vi "randImg.vi"(8 "error in (no error)":errorcluster) -> (0 "error out":errorcluster, 2 "2D Picture":picture, 3 "string out (base64-encoded)":string)   [LabVIEW 2018]
uses:
  abde8a46-2864-4d9c-bf4c-91a7911b97bf.vi
  <vilib>/wsapi/NI_WebServices.lvlib
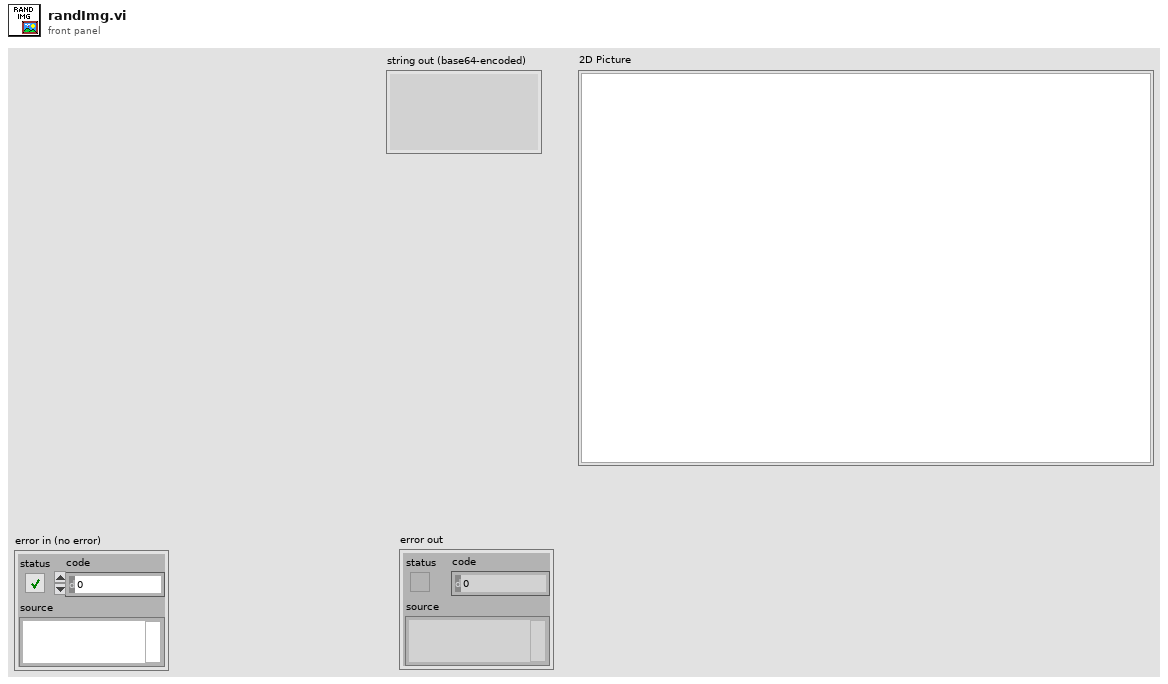
[diagram p1: front panel]
types:
  T1 = typedef "imagedata.ctl" = cluster{"image type":i32, "image depth":i32, "image":u8[], "mask":u8[], "colors":u32[], "Rectangle":cluster{"left":i16, "top":i16, "right":i16, "bottom":i16}}
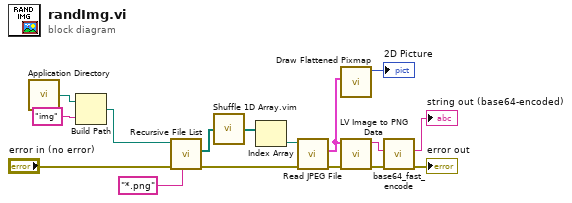
[diagram p0: block diagram]
diagram:
  n1 = call <vilib>:"Application Directory.vi"() -> ("Application Directory"=w10:path)
  n2 = Build Path(base path=w10, name or relative path="img") -> (appended path=w8:path)
  n3 = call <vilib>:"Recursive File List.vi"("pattern"="*.png", "error in (no error)"="error in (no error)", "Folder Path"=w8) -> ("error out"=w11:errorcluster, "All Files in Dir"=w15:path[])  [unwired: 4 in, 3 out]
  n4 = call "Shuffle 1D Array.vim"("array"=w15) -> ("shuffled array"=w14:path[])  [unwired: 4 in]
  n5 = Index Array(array=w14) -> (element=w13:path)  [unwired: 1 in]
  n6 = call <vilib>:"Read JPEG File.vi"("error in (no error)"=w11, "path to JPEG file"=w13) -> ("error out"=w12:errorcluster, "image data"=w3:T1)  [unwired: 7 in, 1 out]
  n7 = call <vilib>:"Draw Flattened Pixmap.vi"("image data"=w3) -> ("new picture"=→"2D Picture":picture)  [unwired: 8 in]
  n8 = call <vilib>:"LV Image to PNG Data.vi"("error in (no error)"=w12, "image data"=w3) -> ("error out"=w7:errorcluster, "png data"=w6:string)  [unwired: 8 in]
  n9 = call "base64_fast_encode.vi"("error in (no error)"=w7, "string in (not encoded)"=w6) -> ("error out"=→"error out":errorcluster, "string out (base64-encoded)"=→"string out (base64-encoded)":string)  [unwired: 8 in]
